vi "MultiTauCorrelationNew.vi"(6 "zero lag +":i32=1, 9 "AC final pts":i64=64, 10 "counts":dbl[](array[numeric]), 11 "First Call":i32=2) -> (2 "Mean of  Bins":dbl format="%0.2f", 3 "Data out":dbl[][](array[numeric]))   [LabVIEW 2022 SP3]
uses:
  <vilib>/Analysis/baseanly.llb/Mean (DBL).vi
  <vilib>/Analysis/NI_AALBase.lvlib
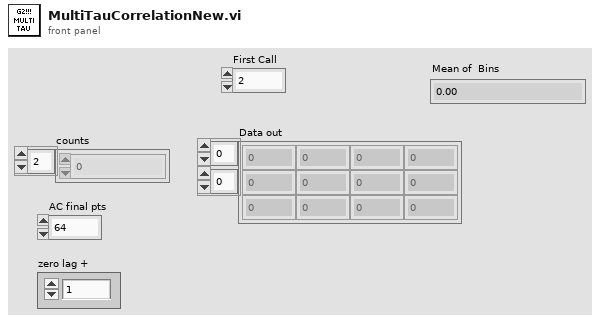
[diagram p1: front panel]
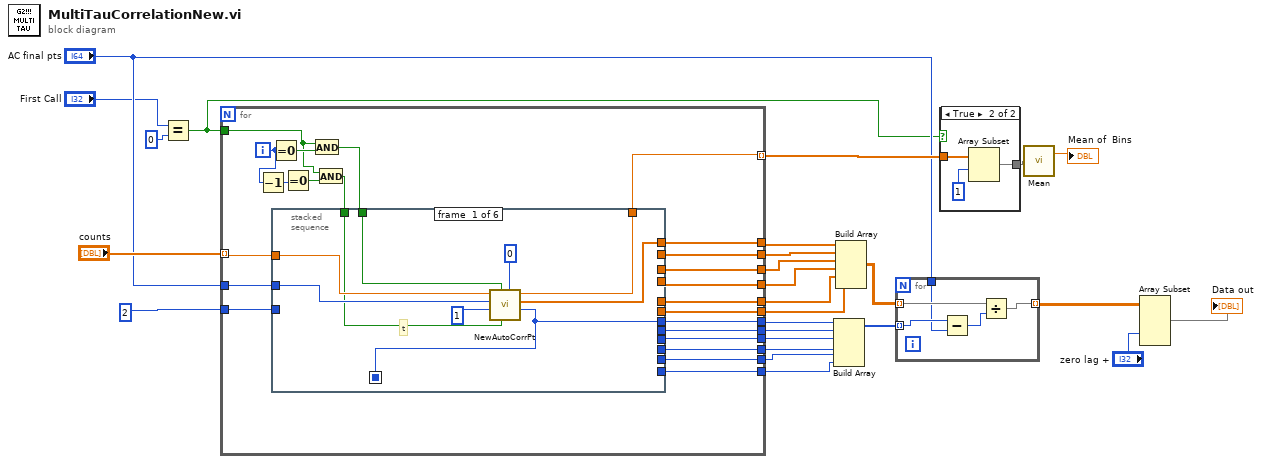
[diagram p0: block diagram]
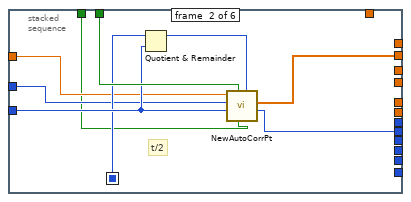
[diagram p3: hidden frame]
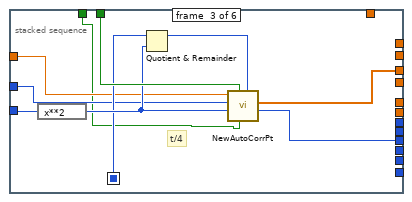
[diagram p4: hidden frame]
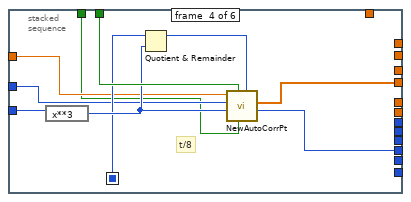
[diagram p5: hidden frame]
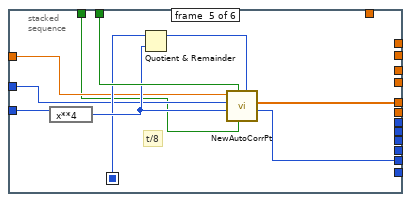
[diagram p6: hidden frame]
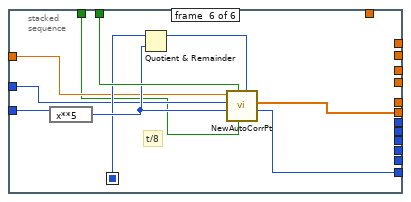
[diagram p7: hidden frame]
diagram:
  n1 = Equal?(x="First Call", y=0) -> (x = y?=w1:bool)
  n2 = for {
    tunnel: "counts" -> [w47] mode=indexing
    tunnel: "AC final pts" -> [w46]
    tunnel: [w40] -> w19
    tunnel: [w39] -> w15
    tunnel: 2 -> [w45]
    tunnel: [w38] -> w23 mode=indexing
    tunnel: [w49] -> w18
    tunnel: [w48] -> w14
    tunnel: [w44] -> w16
    tunnel: [w43] -> w13
    tunnel: [w42] -> w17
    tunnel: [w41] -> w12
    tunnel: [w37] -> w7
    tunnel: [w36] -> w6
    tunnel: [w35] -> w5
    tunnel: [w34] -> w4
    tunnel: w1 -> [w31]
    i -> [w30]
    n3 = Decrement(x=w30) -> (x-1=w29:i32)
    n4 = Equal To 0?(x=w30) -> (x = 0?=w33:bool)
    n5 = Equal To 0?(x=w29) -> (x = 0?=w28:bool)
    n6 = And(x=w31, y=w33) -> (x .and. y?=w32:bool)
    n7 = And(x=w31, y=w28) -> (x .and. y?=w27:bool)
    n8 = stacked-sequence {
      seq-local: [w54 _ _ _ _ _] -> [_ w63 w71 w83 w93 w103]
      tunnel: [_ w62 _ _ _ _] -> w49
      tunnel: [_ w67 _ _ _ _] -> w48
      tunnel: w32 -> [w58 w65 w76 w86 w96 w106]
      tunnel: w47 -> [w52 w61 w70 w81 w92 w102]
      tunnel: w46 -> [w51 w60 w69 w80 w91 w101]
      tunnel: w45 -> [_ w64 w73 w85 w95 w105]
      tunnel: [_ _ w75 _ _ _] -> w44
      tunnel: [_ _ w74 _ _ _] -> w43
      tunnel: [_ _ _ w79 _ _] -> w42
      tunnel: [_ _ _ w82 _ _] -> w41
      tunnel: [w55 _ _ _ _ _] -> w40
      tunnel: [w54 _ _ _ _ _] -> w39
      tunnel: [w53 _ _ _ _ _] -> w38
      tunnel: [_ _ _ _ w90 _] -> w37
      tunnel: [_ _ _ _ w89 _] -> w36
      tunnel: [_ _ _ _ _ w99] -> w35
      tunnel: [_ _ _ _ _ w100] -> w34
      tunnel: w27 -> [w50 w59 w68 w78 w88 w98]
      frame #0 {
        # "t"
        n9 = call "NewAutoCorrPt.vi"("Modulo"=i64 0 ("x-y*floor(x/y)"), "Second?"=w50, "First?"=w58, "divisor"=i64 1 ("x-y*floor(x/y)"), "AC final pts"=w51, "New Count"=w52) -> ("interation out"=w54:i64, "G2 out"=w55:dbl[], "bin out"=w53:dbl)  [unwired: 3 in]
      }
      frame #1 {
        # "t/2"
        n10 = Quotient & Remainder(x=w63, y=w64) -> (x-y*floor(x/y)=w66:i64)  [unwired: 1 out]
        n11 = call "NewAutoCorrPt.vi"("Modulo"=w66, "Second?"=w59, "First?"=w65, "divisor"=w64, "AC final pts"=w60, "New Count"=w61) -> ("interation out"=w67:i64, "G2 out"=w62:dbl[])  [unwired: 3 in, 1 out]
      }
      frame #2 {
        # "t/4"
        n12 = expression code="x**2"(w73) -> (w72:i32)
        n13 = Quotient & Remainder(x=w71, y=w72) -> (x-y*floor(x/y)=w77:i64)  [unwired: 1 out]
        n14 = call "NewAutoCorrPt.vi"("Modulo"=w77, "Second?"=w68, "First?"=w76, "divisor"=w72, "AC final pts"=w69, "New Count"=w70) -> ("interation out"=w74:i64, "G2 out"=w75:dbl[])  [unwired: 3 in, 1 out]
      }
      frame #3 {
        # "t/8"
        n15 = expression code="x**3"(w85) -> (w84:i32)
        n16 = Quotient & Remainder(x=w83, y=w84) -> (x-y*floor(x/y)=w87:i64)  [unwired: 1 out]
        n17 = call "NewAutoCorrPt.vi"("Modulo"=w87, "Second?"=w78, "First?"=w86, "divisor"=w84, "AC final pts"=w80, "New Count"=w81) -> ("interation out"=w82:i64, "G2 out"=w79:dbl[])  [unwired: 3 in, 1 out]
      }
      frame #4 {
        # "t/8"
        n18 = expression code="x**4"(w95) -> (w94:i32)
        n19 = Quotient & Remainder(x=w93, y=w94) -> (x-y*floor(x/y)=w97:i64)  [unwired: 1 out]
        n20 = call "NewAutoCorrPt.vi"("Modulo"=w97, "Second?"=w88, "First?"=w96, "divisor"=w94, "AC final pts"=w91, "New Count"=w92) -> ("interation out"=w89:i64, "G2 out"=w90:dbl[])  [unwired: 3 in, 1 out]
      }
      frame #5 {
        # "t/8"
        n21 = expression code="x**5"(w105) -> (w104:i32)
        n22 = Quotient & Remainder(x=w103, y=w104) -> (x-y*floor(x/y)=w107:i64)  [unwired: 1 out]
        n23 = call "NewAutoCorrPt.vi"("Modulo"=w107, "Second?"=w98, "First?"=w106, "divisor"=w104, "AC final pts"=w101, "New Count"=w102) -> ("interation out"=w99:i64, "G2 out"=w100:dbl[])  [unwired: 3 in, 1 out]
      }
    }
  }
  n24 = Build Array(w15, w14, w13, w12, w6, w5) -> (w11:i64[])
  n25 = Build Array(w19, w18, w16, w17, w7, w4) -> (w10:dbl[][])
  n26 = for {
    tunnel: w11 -> [w110] mode=indexing
    tunnel: w10 -> [w111] mode=indexing
    tunnel: "AC final pts" -> [w109]
    tunnel: [w108] -> w8 mode=indexing
    n27 = Subtract(x=w110, y=w109) -> (x-y=w112:i64)
    n28 = Divide(x=w111, y=w112) -> (x/y=w108:dbl[])
  }
  n29 = case shown="True" w1 {
    tunnel: w23 -> [w113 w116]
    tunnel: [w113 w115] -> w22
    frame False {
    }
    frame True {
      n30 = Array Subset(array=w116, index=1) -> (w115:dbl[])  [unwired: 1 in]
    }
  }
  n31 = call-poly <vilib>:"Mean.vi"("X"=w22) -> ("mean"=→"Mean of  Bins":dbl)  [unwired: 1 out]
  n32 = Array Subset(array=w8, index (col)="zero lag +") -> (→"Data out":dbl[][])  [unwired: 3 in]
